vi "Keith 7001 Error Query.vi"(0 "GPIB address":string, 1 "error in":T1, 2 "source":string) -> (3 "GPIB address out":string, 4 "messages":string, 5 "error out":T1)   [LabVIEW 2019]
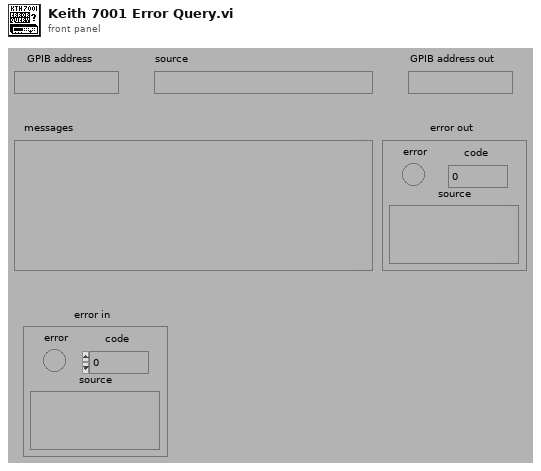
[diagram p1: front panel]
types:
  T1 = cluster{"error":bool, "code":i32, "source":string}
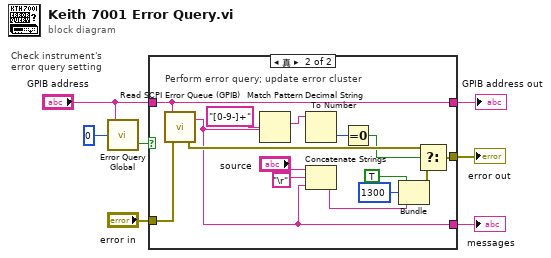
[diagram p0: block diagram]
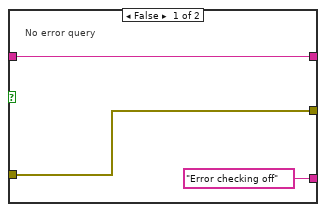
[diagram p2: hidden frame]
diagram:
  # "Check instrument's\nerror query setting"
  n1 = call "Error Query Global.vi"("mode (0:read value)"=u16 0, "GPIB address"="GPIB address") -> ("current setting"=w1:bool)  [unwired: 1 in, 1 out]
  n2 = case shown="真" w1 {
    tunnel: "GPIB address" -> [w8 w14]
    tunnel: "error in" -> [w10 w21]
    tunnel: [w10 w17] -> w3
    tunnel: ["Error checking off" w12] -> w7
    tunnel: [w8 w14] -> w2
    frame False {
      # "No error query"
    }
    frame True {
      # "Perform error query; update error cluster"
      n3 = call "Read SCPI Error Queue (GPIB).vi"("error in"=w21, "GPIB address"=w14) -> ("error out"=w19:T1, "messages"=w12:string)
      n4 = Match Pattern(string=w12, regular expression="[0-9-]+") -> (match substring=w11:string)  [unwired: 1 in, 3 out]
      n5 = Decimal String To Number(string=w11) -> (number=w25:i32)  [unwired: 2 in, 1 out]
      n6 = Concatenate Strings("source", "\r", w12) -> (w22:string)
      n7 = Equal To 0?(x=w25) -> (x = 0?=w18:bool)
      n8 = Bundle(TRUE, 1300, w22) -> (w20:errorcluster)  [unwired: 1 in]
      n9 = Select(t=w19, s=w18, f=w20) -> (s? t:f=w17:T1)
    }
  }
  "messages" <- w7
  "error out" <- w3
  "GPIB address out" <- w2
